vi "AWS-S3-BucketSetPolicy.vi"(0 "AWS-S3-API":refnum<class "AWS-S3-API.lvclass">, 5 "Bucket Name":string, 7 "Policy Document":string, 11 "error in":errorcluster) -> (4 "AWS-S3-API out":refnum<class "AWS-S3-API.lvclass">, 15 "error out":errorcluster)   [LabVIEW 2012, in "AWS-S3-API.lvclass"]
uses:
  AWS-S3-API.lvclass
  C:/Users/Jack/repo/visualize/Dependencies/aws/AWS-SDK/AWSSDK.dll
  AWS-SDK/AWSSDK.dll
panel:
  # "Inputs"
  # "Outputs"
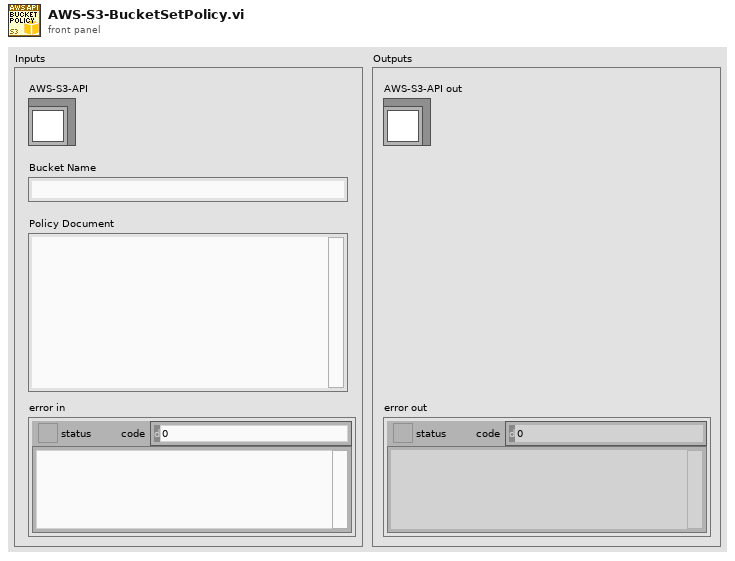
[diagram p1: front panel]
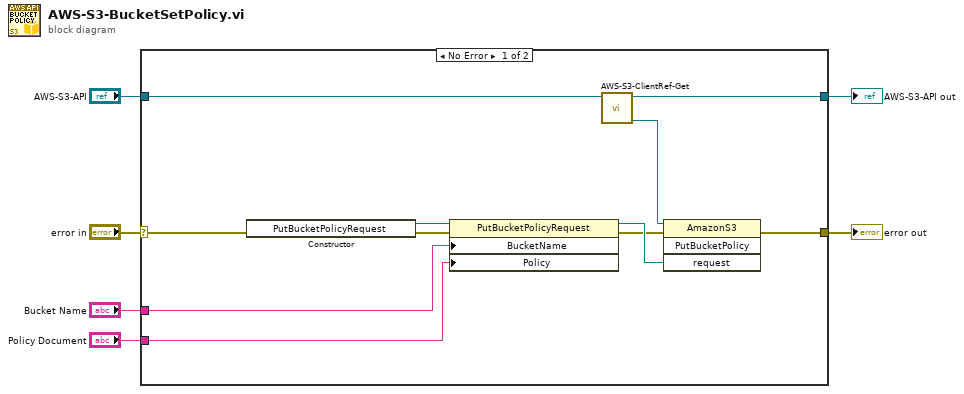
[diagram p0: block diagram]
diagram:
  n1 = case shown="No Error" "error in" {
    selector: "error in" -> [w15 w19]
    tunnel: [w10 w19] -> w6
    tunnel: [w7 w18] -> w4
    tunnel: "AWS-S3-API" -> [w8 w18]
    tunnel: "Bucket Name" -> [w14 _]
    tunnel: "Policy Document" -> [w12 _]
    frame No Error {
      n2 = constructor class="PutBucketPolicyRequest"(error in=w15) -> (reference out=w13:refnum<k24>, error out=w17:errorcluster)  [unwired: 2 in, 1 out]
      n3 = property class="PutBucketPolicyRequest"(reference=w13, error in=w17, "BucketName"=w14, "Policy"=w12) -> (reference out=w16:refnum<k24>, error out=w11:errorcluster)
      n4 = call "AWS-S3-ClientRef-Get.vi"("AWS-S3-API"=w8) -> ("S3 Client ref"=w9:refnum<k24>, "AWS-S3-API out"=w7:refnum<class "AWS-S3-API.lvclass">)  [unwired: 9 in]
      n5 = invoke class="AmazonS3" method="PutBucketPolicy"(reference=w9, error in=w11, "request"=w16) -> (error out=w10:errorcluster)  [unwired: 1 in, 3 out]
    }
    frame Error {
    }
  }
  "error out" <- w6
  "AWS-S3-API out" <- w4
